vi "Hash String to Numeric.vi"(6 "Hash Array":string[][](array[string])=[["I", "1"], ["V", "5"], ["X", "10"], ["L", "50"], ["C", "100"], ["D", "500"], ["M", "1000"]], 8 "error in (no error)":errorcluster, 11 "String Input":string) -> (0 "error out":errorcluster, 3 "Numeric Output":dbl)   [LabVIEW 2023]
doc: "Take in a 2D array as a hashmap(?) and output the string to numeric conversion based on that hashmap"
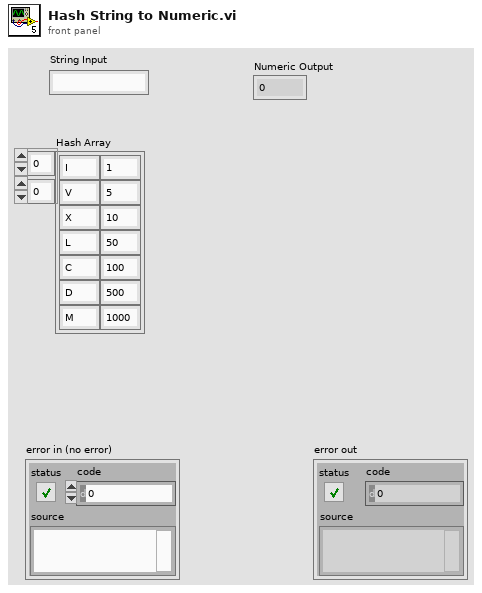
[diagram p1: front panel]
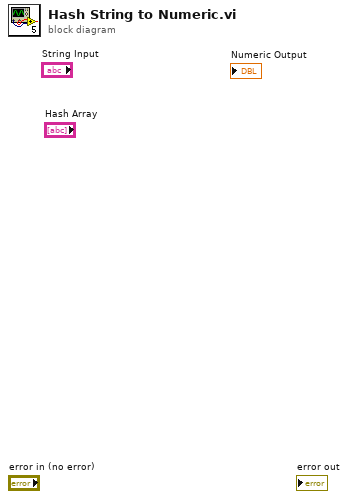
[diagram p0: block diagram]
diagram:
